vi "Get Velocity Setpoint.vi"(8 "error in (no error)":errorcluster, 11 "KUKA youBot wheel motor_EtherCAT in":refnum<class "NI_Robotics_KUKA youBot Wheel Motor_EtherCAT.lvclass">) -> (0 "error out":errorcluster, 2 "CCW velocity (rad/s)":dbl, 3 "KUKA youBot wheel motor_EtherCAT out":refnum<class "NI_Robotics_KUKA youBot Wheel Motor_EtherCAT.lvclass">)   [LabVIEW 2017, in "NI_Robotics_KUKA youBot Host.lvlib" / "NI_Robotics_KUKA youBot Wheel Motor_EtherCAT.lvclass"]
uses:
  <vilib>/robotics/KUKA youBot/Motor/Wheel Motor EtherCAT/NI_Robotics_KUKA youBot Wheel Motor_EtherCAT.lvclass
  <vilib>/robotics/KUKA youBot/Motor/Wheel Motor EtherCAT/NI_Robotics_KUKA youBot Wheel Motor_EtherCAT.lvclass/NI_Robotics_KUKA youBot Wheel Motor_EtherCAT.ctl
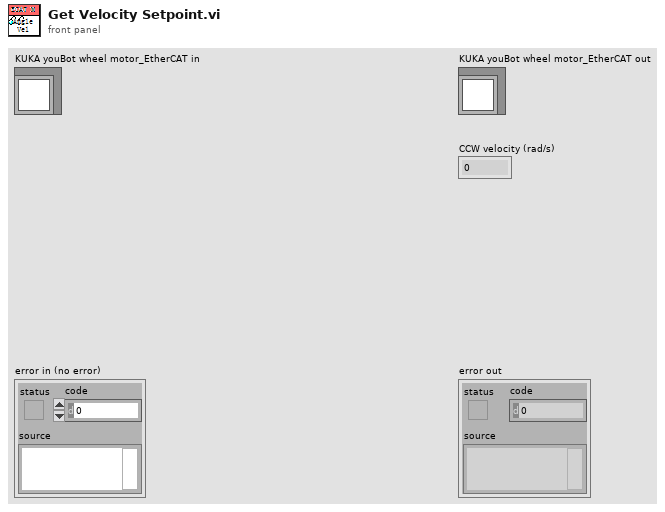
[diagram p1: front panel]
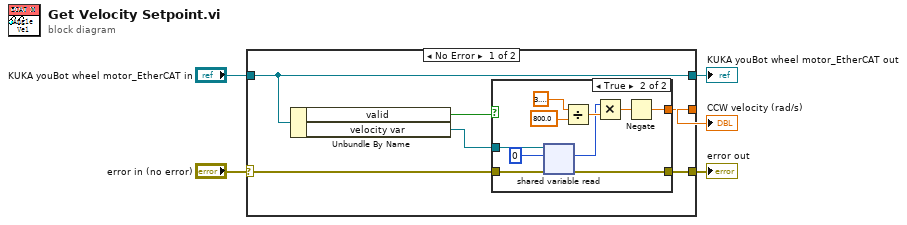
[diagram p0: block diagram]
diagram:
  n1 = case shown="No Error" "error in (no error)" {
    selector: "error in (no error)" -> [w10 w23]
    tunnel: "KUKA youBot wheel motor_EtherCAT in" -> [w9 w24]
    tunnel: [w9 w24] -> w2
    tunnel: [w8 w23] -> w1
    tunnel: [w7 _] -> w3
    frame No Error {
      n2 = Unbundle By Name(w9) -> ("valid"=w6:bool, "velocity var"=w11:refnum<k21>)
      n3 = case shown="True" w6 {
        tunnel: w11 -> [_ w21]
        tunnel: w10 -> [w12 w20]
        tunnel: [w12 w19] -> w8
        tunnel: [_ w13] -> w7
        frame False {
        }
        frame True {
          n4 = shared-variable-read(w21, w20, 0 ("data type")) -> (w19:errorcluster, w14:i32)  [unwired: 2 out]
          n5 = Divide(x=3.141592653589793, y=800.0) -> (x/y=w16:dbl)
          n6 = Multiply(x=w14, y=w16) -> (x*y=w15:dbl)
          n7 = Negate(x=w15) -> (-x=w13:dbl)
        }
      }
    }
    frame Error {
    }
  }
  "error out" <- w1
  "KUKA youBot wheel motor_EtherCAT out" <- w2
  "CCW velocity (rad/s)" <- w3
